vi "CD Engine lvlib.vi"(8 "error in (no error)":errorcluster, 9 "Action":T1) -> (0 "error out":errorcluster, 1 "Output":string)   [LabVIEW 2015]
doc: "Constants, which are necessary for the <B>CD Engine library</B> in the generated custom device project."
uses:
  Constants TypDef/CD Engine lvlib.ctl
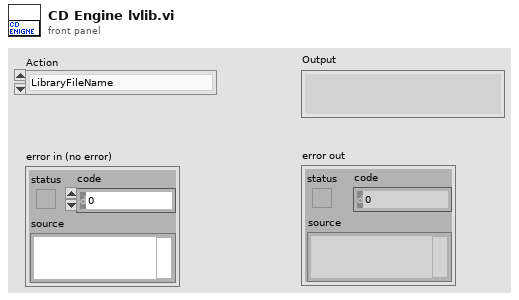
[diagram p1: front panel]
types:
  T1 = typedef "CD Engine lvlib.ctl" = enum16{"LibraryFileName", "LibraryFolderName", "Engine.FolderName", "Engine.Init.FolderName", "Engine.Run.FolderName", "Engine.Shutdown.FolderName", "Types.FolderName", "Engine.RT Driver VI.TemplatePath", "Engine.RT Driver VI.FileName", "Engine.RTStateVariables.Name", "Engine.RTStateVariables.Name.NoExtension", "Engine.Async.NameExtension", "Engine.Async.TemplateName"}
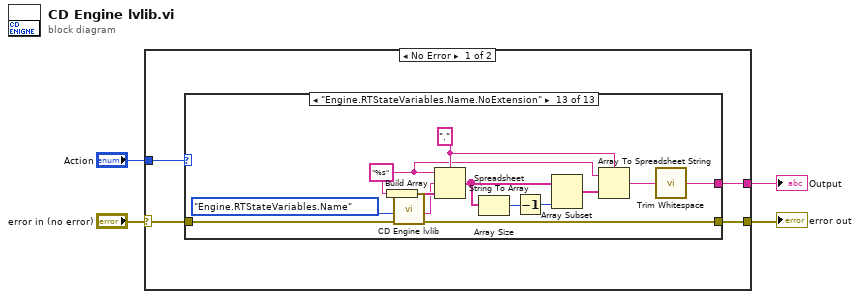
[diagram p0: block diagram]
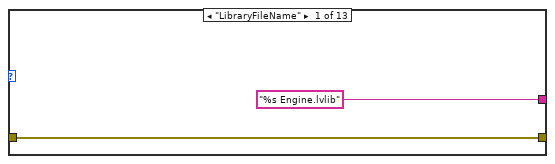
[diagram p2: hidden frame]
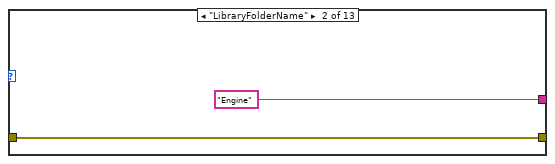
[diagram p3: hidden frame]
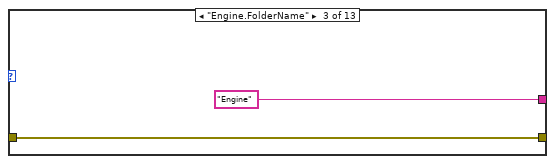
[diagram p4: hidden frame]
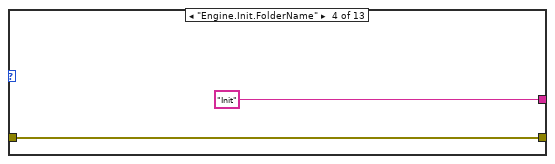
[diagram p5: hidden frame]
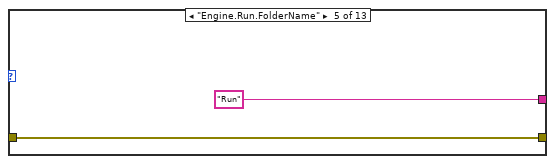
[diagram p6: hidden frame]
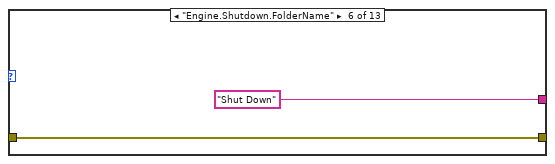
[diagram p7: hidden frame]
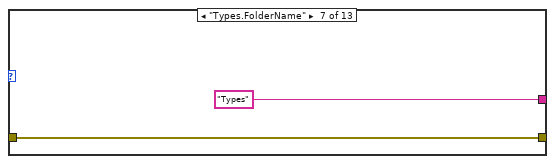
[diagram p8: hidden frame]
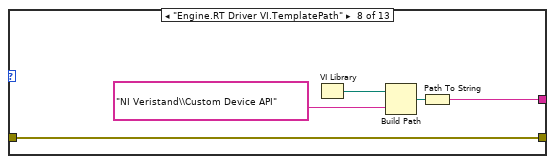
[diagram p9: hidden frame]
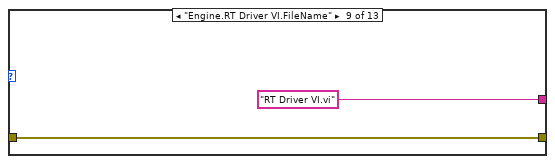
[diagram p10: hidden frame]
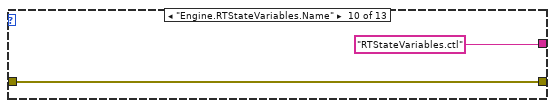
[diagram p11: hidden frame]
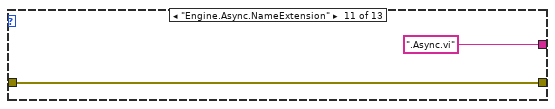
[diagram p12: hidden frame]
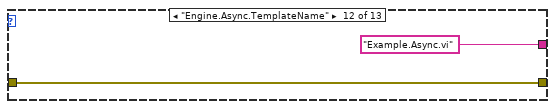
[diagram p13: hidden frame]
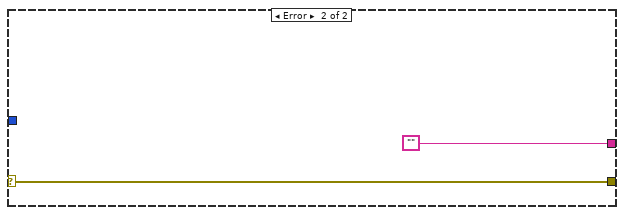
[diagram p14: hidden frame]
diagram:
  n1 = case shown="No Error" "error in (no error)" {
    selector: "error in (no error)" -> [w6 w50]
    tunnel: [w5 w50] -> w1
    tunnel: [w7 ""] -> w2
    tunnel: "Action" -> [w8 _]
    frame No Error {
      n2 = case shown="\"Engine.RTStateVariables.Name.NoExtension\"" w8 {
        tunnel: ["%s Engine.lvlib" "Engine" "Engine" "Init" "Run" "Shut Down" "Types" w24 "RT Driver VI.vi" "RTStateVariables.ctl" ("Output") ".Async.vi" ("name or relative path") "Example.Async.vi" ("name or relative path") w36] -> w7
        tunnel: w6 -> [w9 w11 w13 w15 w17 w19 w21 w23 w28 w30 w32 w34 w40]
        tunnel: [w9 w11 w13 w15 w17 w19 w21 w23 w28 w30 w32 w34 w39] -> w5
        frame "LibraryFileName" {
        }
        frame "LibraryFolderName" {
        }
        frame "Engine.FolderName" {
        }
        frame "Engine.Init.FolderName" {
        }
        frame "Engine.Run.FolderName" {
        }
        frame "Engine.Shutdown.FolderName" {
        }
        frame "Types.FolderName" {
        }
        frame "Engine.RT Driver VI.TemplatePath" {
          n3 = VI Library() -> (path=w25:path)
          n4 = Build Path(base path=w25, name or relative path="NI Veristand\\Custom Device API") -> (appended path=w27:path)
          n5 = Path To String(path=w27) -> (string=w24:string)
        }
        frame "Engine.RT Driver VI.FileName" {
        }
        frame "Engine.RTStateVariables.Name" {
        }
        frame "Engine.Async.NameExtension" {
        }
        frame "Engine.Async.TemplateName" {
        }
        frame "Engine.RTStateVariables.Name.NoExtension" {
          w43 = "." ("delimiter (Tab)")
          w42 = "%s" ("format string")
          n6 = Build Array(w42) -> (w48:string[])
          n7 = call "CD Engine lvlib.vi"("error in (no error)"=w40, "Action"=CD_Engine_lvlib."Engine.RTStateVariables.Name") -> ("error out"=w39:errorcluster, "Output"=w38:string)  [unwired: 8 in]
          n8 = Spreadsheet String To Array(delimiter (Tab)=w43, format string=w42, spreadsheet string=w38, array type (2D Dbl)=w48) -> (array=w47:string[])
          n9 = Array Size(array=w47) -> (size(s)=w46:i32)
          n10 = Decrement(x=w46) -> (x-1=w45:i32)
          n11 = Array Subset(array=w47, length=w45) -> (w44:string[])  [unwired: 1 in]
          n12 = Array To Spreadsheet String(delimiter (Tab)=w43, array=w44, 3:w42) -> (spreadsheet string=w37:string)
          n13 = call <vilib>:"Trim Whitespace.vi"("string"=w37) -> ("trimmed string"=w36:string)  [unwired: 1 in]
        }
      }
    }
    frame Error {
    }
  }
  "error out" <- w1
  "Output" <- w2
